vi "Configure Channel (Com).vi"(0 "VISA resource name":refnum<visa-resource-name>, 5 "Channel (001)":string="001", 7 "Enable Channel (False)":bool, 9 "Span":T1={"Enable Span (False)"=FALSE, "Decimal Place (2)"=2, "Lower Span (0.00)"=0.0, "Upper Span (100.00)"=100.0, "Unit Character (\"\")"=""} {"Upper Span (100.00)" min=-9999999.0 max=99999999.0 format="%#_8g"; "Lower Span (0.00)" min=-9999999.0 max=99999999.0 format="%#_8g"; "Decimal Place (2)" min=0 max=5 step=1}, 11 "error in (no error)":errorcluster) -> (4 "VISA resource name out":refnum<visa-resource-name>, 6 "Channel":string, 15 "error out":errorcluster)   [LabVIEW 2020, in "Yokogawa GX Series.lvlib"]
doc: "Sets the input range of com channels.\n\nCommand: SRangeCom"
uses:
  <instrlib>/Yokogawa GX Series/Yokogawa GX Series.lvlib
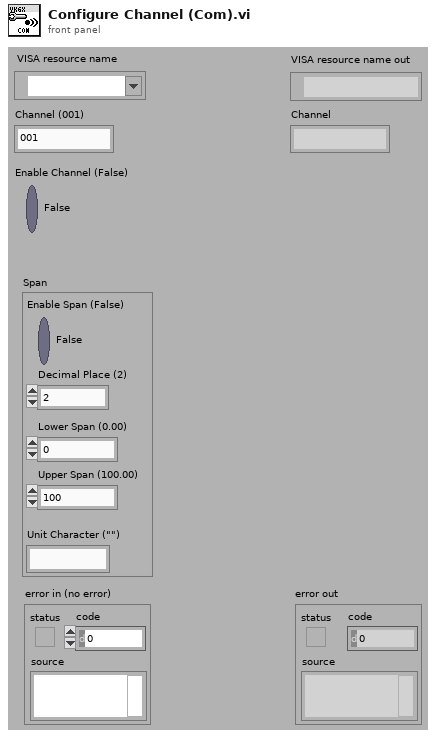
[diagram p1: front panel]
types:
  T1 = cluster{"Enable Span (False)":bool, "Decimal Place (2)":i32, "Lower Span (0.00)":dbl, "Upper Span (100.00)":dbl, "Unit Character (\"\")":string}
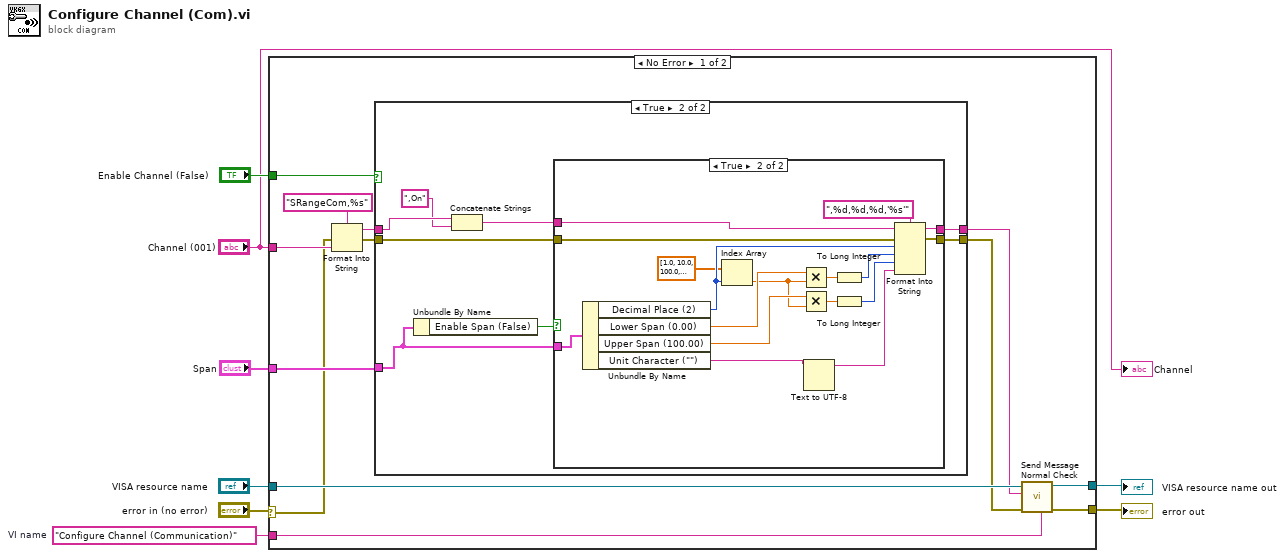
[diagram p0: block diagram]
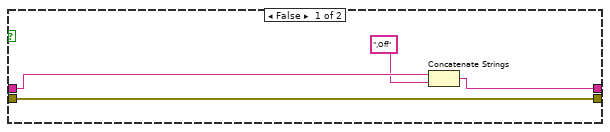
[diagram p2: hidden frame]
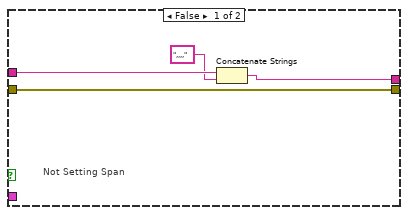
[diagram p3: hidden frame]
diagram:
  w5 = "Configure Channel (Communication)"  # VI name
  n1 = case shown="No Error" "error in (no error)" {
    selector: "error in (no error)" -> [w9 w55]
    tunnel: [w19 w55] -> w8
    tunnel: [w18 w56] -> w7
    tunnel: "VISA resource name" -> [w17 w56]
    tunnel: w5 -> [w14 _]
    tunnel: "Enable Channel (False)" -> [w12 _]
    tunnel: "Channel (001)" -> [w11 _]
    tunnel: "Span" -> [w10 _]
    frame No Error {
      n2 = Format Into String(format string="SRangeCom,%s", error in=w9, w11) -> (resulting string=w13:string, error out=w20:errorcluster)  [unwired: 1 in]
      n3 = case shown="True" w12 {
        tunnel: w20 -> [w22 w29]
        tunnel: w10 -> [_ w31]
        tunnel: [w22 w33] -> w16
        tunnel: [w23 w32] -> w15
        tunnel: w13 -> [w25 w28]
        frame False {
          n4 = Concatenate Strings(w25, ",Off") -> (w23:string)
        }
        frame True {
          n5 = Unbundle By Name(w31) -> ("Enable Span (False)"=w30:bool)
          n6 = Concatenate Strings(w28, ",On") -> (w27:string)
          n7 = case shown="True" w30 {
            tunnel: w29 -> [w37 w53]
            tunnel: [w37 w52] -> w33
            tunnel: w27 -> [w36 w42]
            tunnel: [w34 w51] -> w32
            tunnel: w31 -> [_ w48]
            frame False {
              # "Not Setting Span"
              n8 = Concatenate Strings(w36, ",,,,") -> (w34:string)
            }
            frame True {
              n9 = Unbundle By Name(w48) -> ("Decimal Place (2)"=w45:i32, "Lower Span (0.00)"=w47:dbl, "Upper Span (100.00)"=w46:dbl, "Unit Character (\"\")"=w39:string)
              n10 = Index Array(array=dbl[] [1.0, 10.0, 100.0, 1000.0, 10000.0, 100000.0], index=w45) -> (element=w40:dbl)
              n11 = Multiply(x=w47, y=w40) -> (x*y=w50:dbl)
              n12 = Multiply(x=w46, y=w40) -> (x*y=w49:dbl)
              n13 = Text to UTF-8(11:w39) -> (3:w38:string)  [unwired: 2 in, 1 out]
              n14 = To Long Integer(number=w50) -> (32bit integer=w44:i32)
              n15 = To Long Integer(number=w49) -> (32bit integer=w43:i32)
              n16 = Format Into String(format string=",%d,%d,%d,'%s'", initial string=w42, error in=w53, w45, w44, w43, w38) -> (resulting string=w51:string, error out=w52:errorcluster)
            }
          }
        }
      }
      n17 = call <instrlib>:"Send Message Normal Check.vi"("Source (\"\")"=w14, "error in (no error)"=w16, "Send Message (\"\")"=w15, "VISA resource name"=w17) -> ("error out"=w19:errorcluster, "VISA resource name out"=w18:refnum<visa-resource-name>)  [unwired: 2 in, 4 out]
    }
    frame Error {
    }
  }
  "error out" <- w8
  "VISA resource name out" <- w7
  "Channel" <- "Channel (001)"
